vi "Create Engine Folder and Copy RT Template.vi"(8 "error in":errorcluster, 9 "Project Root":path, 10 "Project Name":string, 11 "CD Template":refnum<class "NIVS_PPL_Inline HW Interface.lvclass">) -> (0 "error out":errorcluster)   [LabVIEW 2020, in "NIVS_PPL_Inline HW Interface.lvclass"]
uses:
  NIVS_PPL_Inline HW Interface.lvclass
  C:/dev/Karthick/FPGA Addons Packages/niveristand-custom-device-wizard/ProjectTemplate/Source/NI VeriStand/Custom Device/Template Classes/NIVS_CD Template/NIVS_CD Template.lvclass
  NIVS_Consolidated_CDW_MetaDataObj/CD Engine lvlib.ctl
  NIVS_Consolidated_CDW_MetaDataObj/Common.ctl
  NIVS_CD Template/NIVS_CD Template.lvclass/NIVS_CD Template.ctl
  NIVS_Consolidated_CDW_MetaDataObj/Common.vi
  NIVS_Consolidated_CDW_MetaDataObj/NIVS_Consolidated_CDW_MetaDataObj.lvclass
  NIVS_CD Template/NIVS_CD Template.lvclass
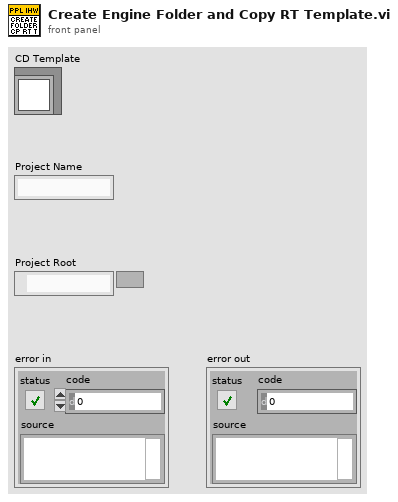
[diagram p1: front panel]
types:
  T1 = typedef "NIVS_Consolidated_CDW_MetaDataObj.lvclass/CD Engine lvlib.ctl" = enum16{"LibraryFileName", "LibraryFolderName", "Engine.FolderName", "Engine.Init.FolderName", "Engine.Run.FolderName", "Engine.Shutdown.FolderName", "Types.FolderName", "Engine.RT Driver VI.TemplatePath", "Engine.RT Driver VI.FileName", "Engine.PPL.RT Driver VI_InlineAsync.FileName", "Engine.RTStateVariables.Name", "Engine.PPL.RTStateVariables.Name", "Engine.RTStateVariables.Name.NoExtension", "Engine.Async.NameExtension", "Engine.Async.TemplateName", "Engine.PPL.Async.TemplateName", "Engine.PPL.Async.InitVSGlobals.Name", "Engine.PPL.RT Driver VI_Inline.FileName", "Engine.LaunchCommandLoop.Name", "Engine.CommandLoop.Name"}
  T2 = typedef "NIVS_Consolidated_CDW_MetaDataObj.lvclass/Common.ctl" = enum16{"ProjectName", "TemplatesFolderName", "PPLTemplatesFolderName", "ProjectTemplatePathAndName", "ProjectPPLTemplatePathAndName", "TimingAndSyncFolderName", "CustomDeviceFolderName", "PathToTemplates", "PathToPPLTemplates", "PathToExplorerPPLTemplates", "PathToEnginePPLTemplates", "PathToConfigurationFile", "ProjectConfigurationName"}
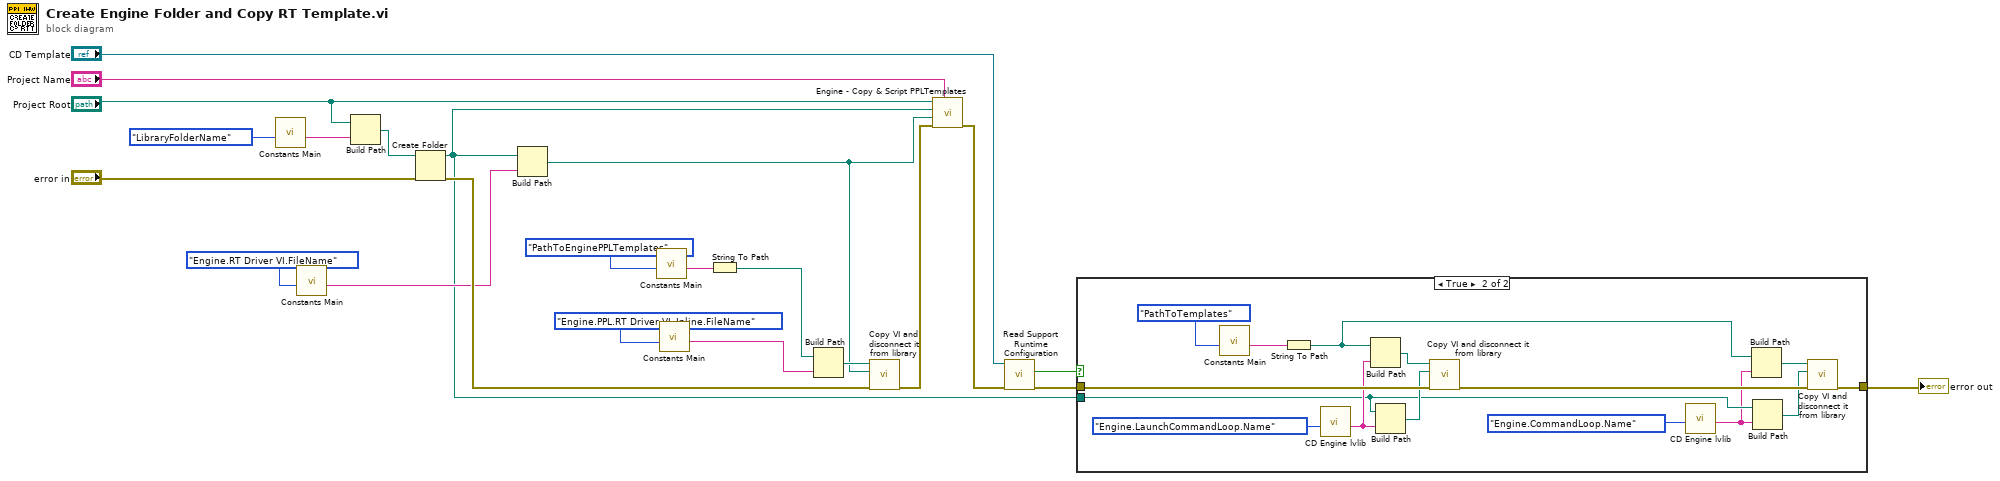
[diagram p0: block diagram]
diagram:
  n1 = call-poly "Constants Main.vi"("Action"=CD_Engine_lvlib."LibraryFolderName") -> ("Output"=w12:string)  [unwired: 10 in]
  n2 = call-poly "Constants Main.vi"("Action"=CD_Engine_lvlib."Engine.RT Driver VI.FileName") -> ("Output"=w8:string)  [unwired: 10 in]
  n3 = Build Path(base path="Project Root", name or relative path=w12) -> (appended path=w14:path)
  n4 = Create Folder(path (use dialog)=w14, error in="error in") -> (created path=w3:path, error out=w22:errorcluster)  [unwired: 1 in, 1 out]
  n5 = Build Path(base path=w3, name or relative path=w8) -> (appended path=w1:path)
  n6 = call-poly "Constants Main.vi"("Action"=Common."PathToEnginePPLTemplates") -> ("Output"=w9:string)  [unwired: 10 in]
  n7 = call-poly "Constants Main.vi"("Action"=CD_Engine_lvlib."Engine.PPL.RT Driver VI_Inline.FileName") -> ("Output"=w16:string)  [unwired: 10 in]
  n8 = String To Path(string=w9) -> (path=w15:path)
  n9 = Build Path(base path=w15, name or relative path=w16) -> (appended path=w10:path)
  n10 = call "Copy VI and disconnect it from library.vi"("error in (no error)"=w22, "VI Target Path"=w1, "VI Source Path"=w10) -> ("error out"=w23:errorcluster)  [unwired: 8 in]
  n11 = call "Engine - Copy & Script PPLTemplates.vi"("CD Name"="Project Name", "error in (no error)"=w23, "RT Driver VI Path"=w1, "RT Driver Folder Path"=w3, "CD Source Folder Path"="Project Root") -> ("error out"=w19:errorcluster)  [unwired: 6 in]
  n12 = call "Read Support Runtime Configuration.vi"("error in"=w19, "NIVS_CD Template in"="CD Template") -> ("error out"=w20:errorcluster, "Support Runtime Configuration"=w2:bool)  [unwired: 7 in, 1 out]
  n13 = case shown="True" w2 {
    tunnel: w20 -> [w24 w39]
    tunnel: [w24 w37] -> w18
    tunnel: w3 -> [_ w29]
    frame False {
    }
    frame True {
      n14 = call-poly "Constants Main.vi"("Action"=Common."PathToTemplates") -> ("Output"=w32:string)  [unwired: 10 in]
      n15 = String To Path(string=w32) -> (path=w26:path)
      n16 = call "CD Engine lvlib.vi"("Action"=CD_Engine_lvlib."Engine.LaunchCommandLoop.Name") -> ("Output"=w31:string)  [unwired: 10 in]
      n17 = Build Path(base path=w26, name or relative path=w31) -> (appended path=w33:path)
      n18 = Build Path(base path=w29, name or relative path=w31) -> (appended path=w35:path)
      n19 = call "Copy VI and disconnect it from library.vi"("error in (no error)"=w39, "VI Target Path"=w35, "VI Source Path"=w33) -> ("error out"=w38:errorcluster)  [unwired: 8 in]
      n20 = call "CD Engine lvlib.vi"("Action"=CD_Engine_lvlib."Engine.CommandLoop.Name") -> ("Output"=w25:string)  [unwired: 10 in]
      n21 = Build Path(base path=w26, name or relative path=w25) -> (appended path=w27:path)
      n22 = Build Path(base path=w29, name or relative path=w25) -> (appended path=w28:path)
      n23 = call "Copy VI and disconnect it from library.vi"("error in (no error)"=w38, "VI Target Path"=w28, "VI Source Path"=w27) -> ("error out"=w37:errorcluster)  [unwired: 8 in]
    }
  }
  "error out" <- w18
